vi "led gradient.vi"() -> ()   [LabVIEW 2019]
uses:
  <vilib>/Rock Robotics/SystemInterfaces/DIO/FPGA_DIOPWMChannel.ctl
panel:
  out "Numeric":i32
  in  "Color Box":u32(colorbox)
  in  "Color Box 2":u32(colorbox)
  out "Color":u32(colorbox)
  out "output array":u32[](array[numeric])
  in  "PWM Channel":T1=enum."PWM 9"
  in  "String Length":u32=8
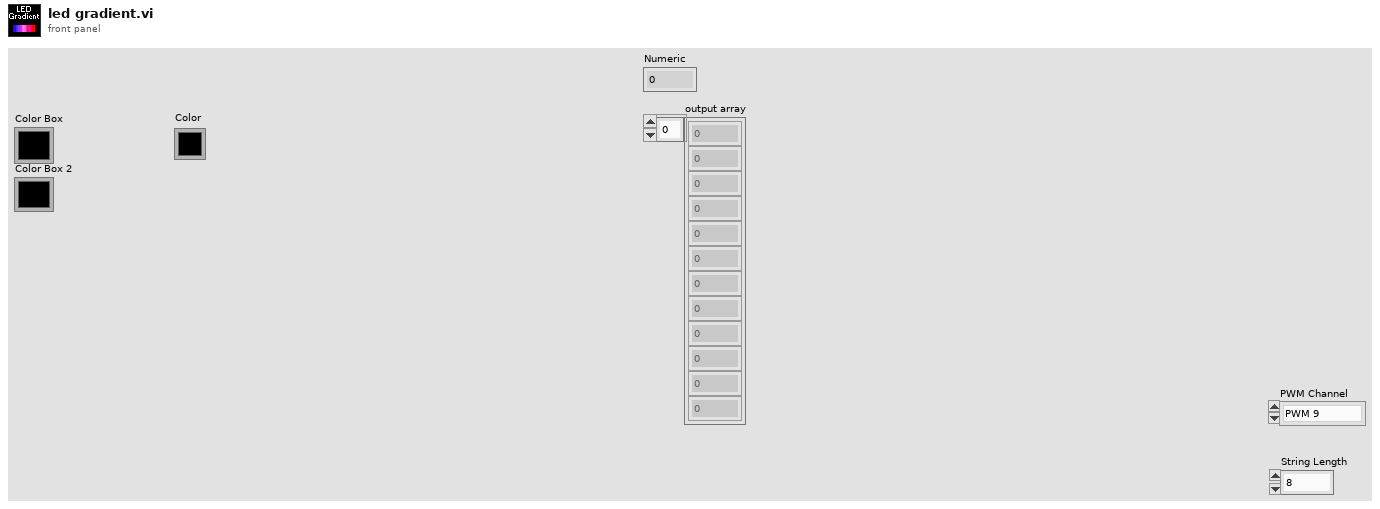
[diagram p1: front panel]
types:
  T1 = typedef "FPGA_DIOPWMChannel.ctl" = enum8{"PWM 0", "PWM 1", "PWM 2", "PWM 3", "PWM 4", "PWM 5", "PWM 6", "PWM 7", "PWM 8", "PWM 9", "PWM MXP 0", "PWM MXP 1", "PWM MXP 2", "PWM MXP 3", "PWM MXP 4", "PWM MXP 5", "PWM MXP 6", "PWM MXP 7", "PWM MXP 8", "PWM MXP 9", "Invalid"}
  T2 = typedef "WPI_PWMDeviceRef.ctl" = cluster{"DeviceStatus":errorcluster, "PWM Channel":T1}
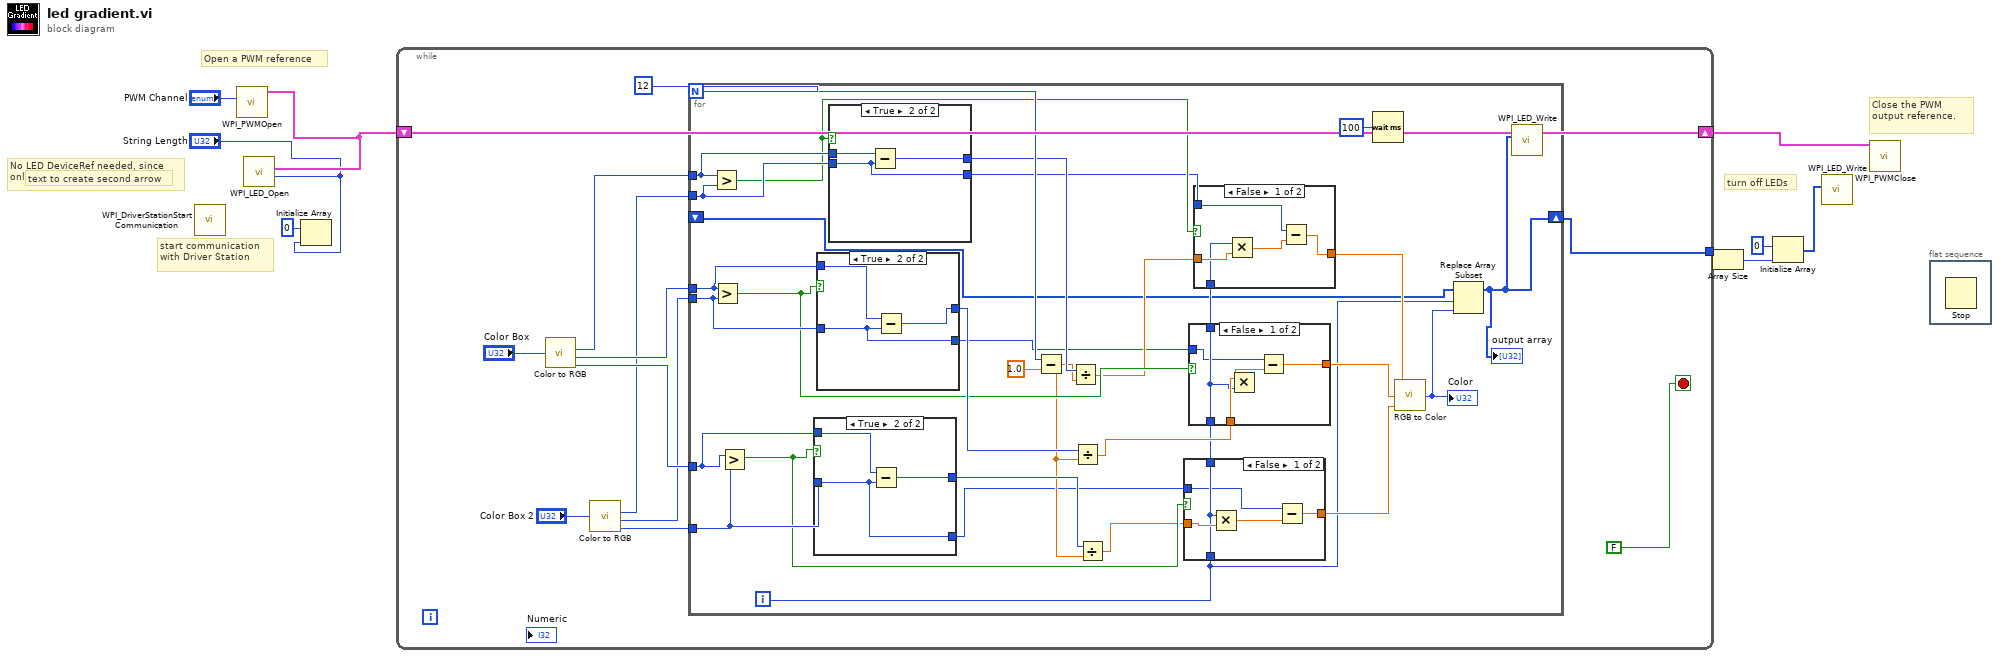
[diagram p0: block diagram]
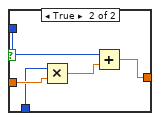
[diagram p2: hidden frame]
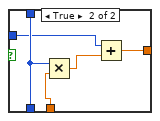
[diagram p3: hidden frame]
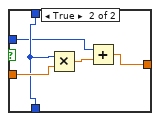
[diagram p4: hidden frame]
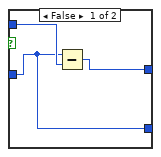
[diagram p5: hidden frame]
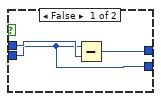
[diagram p6: hidden frame]
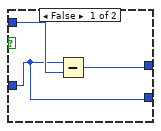
[diagram p7: hidden frame]
diagram:
  # "Open a PWM reference"
  # "start communication with Driver Station"
  # "turn off LEDs"
  # "No LED DeviceRef needed, since only one LED strip is supported"
  # "Close the PWM output reference."
  # "text to create second arrow"
  n1 = call <vilib>:"WPI_DriverStationStart Communication.vi"() -> ()  [unwired: 2 in, 10 out]
  n2 = call <vilib>:"WPI_PWMOpen.vi"("PWM Channel"="PWM Channel") -> ("PWMDeviceRef"=w4:T2)  [unwired: 9 in, 1 out]
  n3 = call <vilib>:"WPI_LED_Open.vi"("String Length"="String Length", "PWMDeviceRef"=w4) -> ()  [unwired: 9 in, 1 out]
  n4 = Initialize Array(u32 0 ("element"), "String Length") -> ()  [unwired: 1 out]
  n5 = while {
    shift-right: [w12] -> w9
    shift-left: w4 -> [w12]
    tunnel: [w10] -> w1
    stop <- FALSE stop-if-true
    n6 = call <vilib>:"Color to RGB.vi"("Color"="Color Box") -> ("R"=w18:u8, "G"=w19:u8, "B"=w17:u8)  [unwired: 1 out]
    n7 = call <vilib>:"Color to RGB.vi"("Color"="Color Box 2") -> ("R"=w14:u8, "G"=w15:u8, "B"=w16:u8)  [unwired: 1 out]
    n8 = for {
      N: 12 -> [w51]
      tunnel: w18 -> [w50]
      tunnel: w19 -> [w47]
      tunnel: w17 -> [w44]
      tunnel: w16 -> [w43]
      tunnel: w15 -> [w46]
      tunnel: w14 -> [w49]
      shift-right: [w22] -> w10
      shift-left: _ -> [w23]
      i -> [w25]
      n9 = Greater?(x=w50, y=w49) -> (0:w41:bool)
      n10 = Greater?(x=w47, y=w46) -> (0:w40:bool)
      n11 = Greater?(x=w44, y=w43) -> (0:w39:bool)
      n12 = case shown="True" w39 {
        tunnel: [w85 w88] -> w45
        tunnel: w44 -> [w84 w87]
        tunnel: w43 -> [w83 w86]
        tunnel: [w83 w86] -> w29
        frame False {
          n13 = Subtract(x=w83, y=w84) -> (x-y=w85:u8)
        }
        frame True {
          n14 = Subtract(x=w87, y=w86) -> (x-y=w88:u8)
        }
      }
      n15 = case shown="True" w40 {
        tunnel: w47 -> [w96 w100]
        tunnel: w46 -> [w95 w98]
        tunnel: [w97 w99] -> w42
        tunnel: [w95 w98] -> w28
        frame False {
          n16 = Subtract(x=w95, y=w96) -> (x-y=w97:u8)
        }
        frame True {
          n17 = Subtract(x=w100, y=w98) -> (x-y=w99:u8)
        }
      }
      n18 = case shown="True" w41 {
        tunnel: w50 -> [w90 w94]
        tunnel: w49 -> [w89 w92]
        tunnel: [w91 w93] -> w48
        tunnel: [w89 w92] -> w27
        frame False {
          n19 = Subtract(x=w89, y=w90) -> (x-y=w91:u8)
        }
        frame True {
          n20 = Subtract(x=w94, y=w92) -> (x-y=w93:u8)
        }
      }
      n21 = Subtract(x=w51, y=1.0) -> (x-y=w30:dbl)
      n22 = Divide(x=w48, y=w30) -> (x/y=w36:dbl)
      n23 = Divide(x=w42, y=w30) -> (x/y=w37:dbl)
      n24 = Divide(x=w45, y=w30) -> (x/y=w38:dbl)
      n25 = case shown="False" w39 {
        tunnel: w38 -> [w76 w80]
        tunnel: [w77 w81] -> w35
        tunnel: w25 -> [w74 w79]
        tunnel: [w74 w79] -> w32
        tunnel: w29 -> [w73 w78]
        frame False {
          n26 = Multiply(x=w74, y=w76) -> (x*y=w75:dbl)
          n27 = Subtract(x=w73, y=w75) -> (x-y=w77:dbl)
        }
        frame True {
          n28 = Multiply(x=w79, y=w80) -> (x*y=w82:dbl)
          n29 = Add(x=w78, y=w82) -> (x+y=w81:dbl)
        }
      }
      n30 = case shown="False" w40 {
        tunnel: w37 -> [w65 w71]
        tunnel: [w67 w69] -> w33
        tunnel: w32 -> [w64 w70]
        tunnel: [w64 w70] -> w31
        tunnel: w28 -> [w63 w68]
        frame False {
          n31 = Multiply(x=w65, y=w64) -> (x*y=w66:dbl)
          n32 = Subtract(x=w63, y=w66) -> (x-y=w67:dbl)
        }
        frame True {
          n33 = Multiply(x=w70, y=w71) -> (x*y=w72:dbl)
          n34 = Add(x=w68, y=w72) -> (x+y=w69:dbl)
        }
      }
      n35 = case shown="False" w41 {
        tunnel: w36 -> [w55 w61]
        tunnel: [w57 w59] -> w34
        tunnel: w31 -> [w54 w60]
        tunnel: w27 -> [w53 w58]
        frame False {
          n36 = Multiply(x=w54, y=w55) -> (x*y=w56:dbl)
          n37 = Subtract(x=w53, y=w56) -> (x-y=w57:dbl)
        }
        frame True {
          n38 = Multiply(x=w60, y=w61) -> (x*y=w62:dbl)
          n39 = Add(x=w58, y=w62) -> (x+y=w59:dbl)
        }
      }
      n40 = Wait (ms)(milliseconds to wait=u32 100) -> ()  [unwired: 1 out]
      n41 = call <vilib>:"RGB to Color.vi"("B"=w35, "G"=w33, "R"=w34) -> ("Color"=w26:u32)
      "Color" <- w26
      n42 = Replace Array Subset(array=w23, new element=w26, index=w25) -> (w22:u32[])
      "output array" <- w22
      n43 = call <vilib>:"WPI_LED_Write.vi"("Color Array"=w22) -> ()  [unwired: 10 in, 1 out]
    }
  }
  n44 = Array Size(array=w1) -> (size(s)=w8:i32)
  n45 = Initialize Array(u32 0, w8) -> (w6:u32[])
  n46 = call <vilib>:"WPI_LED_Write.vi"("Color Array"=w6) -> ()  [unwired: 10 in, 1 out]
  n47 = call <vilib>:"WPI_PWMClose.vi"("PWMDeviceRef"=w9) -> ()  [unwired: 10 in, 1 out]
  n48 = flat-sequence {
    frame #0 {
      n49 = Stop() -> ()  [unwired: 1 in]
    }
  }
